vi "recursive_set_cluster_element.vi"   [LabVIEW 2015]
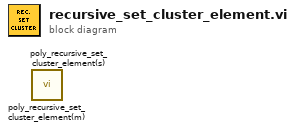
[diagram p0: block diagram]
diagram:
  n1 = call "poly_recursive_set_cluster_element(m).vi"() -> ()  [unwired: 9 in, 3 out]
  n2 = call "poly_recursive_set_cluster_element(s).vi"() -> ()  [unwired: 9 in, 3 out]
